vi "DriveAutoArc.vi"(5 "Forward/Reverse":enum16{"Forward", "Reverse"}(ring), 6 "Use Distance?":bool=TRUE, 7 "Right/Left":enum16{"Right/CW", "Left/CCW"}(ring), 8 "End value (dist or angle)":dbl, 11 "Arc Difference":dbl) -> (0 "Done?":bool, 2 "Right Drive Value":dbl, 3 "Left Drive Value":dbl)   [LabVIEW 2017, in "AutoDrive.lvclass"]
uses:
  AutoSubsystem/AutoDrive/AutoDrive.lvclass
  SensorDataGlobal.vi
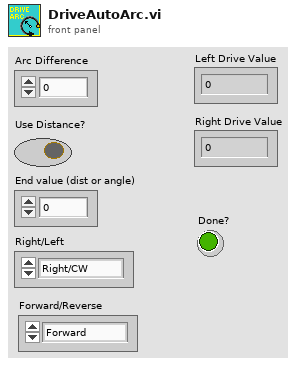
[diagram p1: front panel]
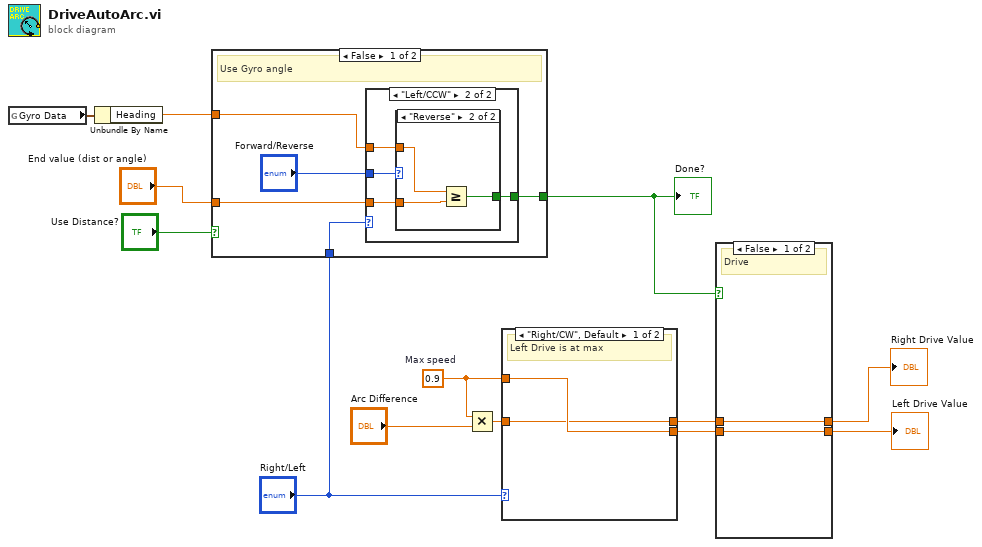
[diagram p0: block diagram]
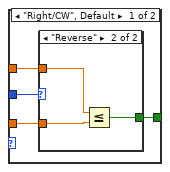
[diagram p2: hidden frame]
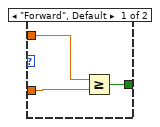
[diagram p3: hidden frame]
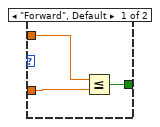
[diagram p4: hidden frame]
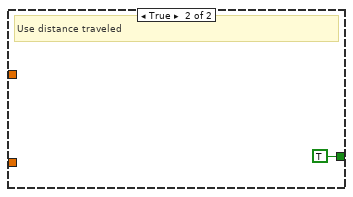
[diagram p5: hidden frame]
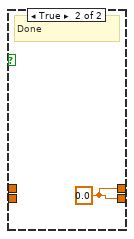
[diagram p7: hidden frame]
diagram:
  w10 = 0.9  # Max speed
  n1 = global read "SensorDataGlobal.vi" "Gyro Data"() -> (w3:cluster{"Heading":dbl, "Gyro Raw":dbl})
  n2 = Unbundle By Name(w3) -> ("Heading"=w2:dbl)
  n3 = case shown="False" "Use Distance?" {
    tunnel: [w18 TRUE] -> w5
    tunnel: "End value (dist or angle)" -> [w15 _]
    tunnel: w2 -> [w16 _]
    tunnel: "Right/Left" -> [w14 _]
    frame False {
      # "Use Gyro angle"
      n4 = case shown="\"Left/CCW\"" w14 {
        tunnel: [w22 w32] -> w18
        tunnel: "Forward/Reverse" -> [w19 w31]
        tunnel: w16 -> [w21 w30]
        tunnel: w15 -> [w20 w29]
        frame "Right/CW", Default {
          n5 = case shown="\"Reverse\"" w19 {
            tunnel: [w23 w28] -> w22
            tunnel: w21 -> [w25 w27]
            tunnel: w20 -> [w24 w26]
            frame "Forward", Default {
              n6 = Greater Or Equal?(x=w25, y=w24) -> (x >= y?=w23:bool)
            }
            frame "Reverse" {
              n7 = Less Or Equal?(x=w27, y=w26) -> (x <= y?=w28:bool)
            }
          }
        }
        frame "Left/CCW" {
          n8 = case shown="\"Reverse\"" w31 {
            tunnel: [w33 w38] -> w32
            tunnel: w30 -> [w35 w37]
            tunnel: w29 -> [w34 w36]
            frame "Forward", Default {
              n9 = Less Or Equal?(x=w35, y=w34) -> (x <= y?=w33:bool)
            }
            frame "Reverse" {
              n10 = Greater Or Equal?(x=w37, y=w36) -> (x >= y?=w38:bool)
            }
          }
        }
      }
    }
    frame True {
      # "Use distance traveled"
    }
  }
  "Done?" <- w5
  n11 = Multiply(x=w10, y="Arc Difference") -> (x*y=w7:dbl)
  n12 = case shown="\"Right/CW\", Default" "Right/Left" {
    tunnel: [w40 w43] -> w11
    tunnel: w10 -> [w41 w43]
    tunnel: [w41 w42] -> w8
    tunnel: w7 -> [w40 w42]
    frame "Right/CW", Default {
      # "Left Drive is at max"
    }
    frame "Left/CCW" {
      # "Right Drive is at max"
    }
  }
  n13 = case shown="False" w5 {
    tunnel: [w45 w46] -> w12
    tunnel: [w44 w46] -> w13
    tunnel: w11 -> [w45 _]
    tunnel: w8 -> [w44 _]
    frame False {
      # "Drive"
    }
    frame True {
      w46 = 0.0
      # "Done"
    }
  }
  "Left Drive Value" <- w13
  "Right Drive Value" <- w12
